vi "Launch Dynamically Load Graphics.vi"(4 "User events":T1, 6 "Template saved?":bool, 7 "Path":T2=enum."Glyphs", 8 "error in (no error)":errorcluster, 10 "button ref":refnum<vi>, 11 "animatedDecoration ref":refnum<vi>) -> (0 "error out":errorcluster)   [LabVIEW 2020]
uses:
  vi.lib/LabVIEW Icon API/lv_icon/lv_icon.lvlib
  vi.lib/LabVIEW Icon API/lv_icon/Controls/Pathes.ctl
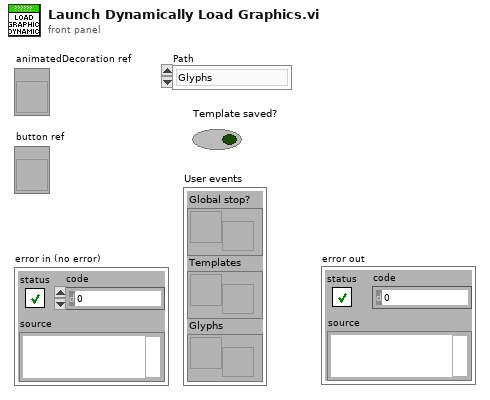
[diagram p1: front panel]
types:
  T1 = cluster{"Global stop?":refnum<user-event>, "Templates":refnum<user-event>, "Glyphs":refnum<user-event>}
  T2 = typedef "Pathes.ctl" = enum16{"Root Path", "Icon Templates", "Icon Templates VI", "Icon Templates Lib", "Glyphs"}
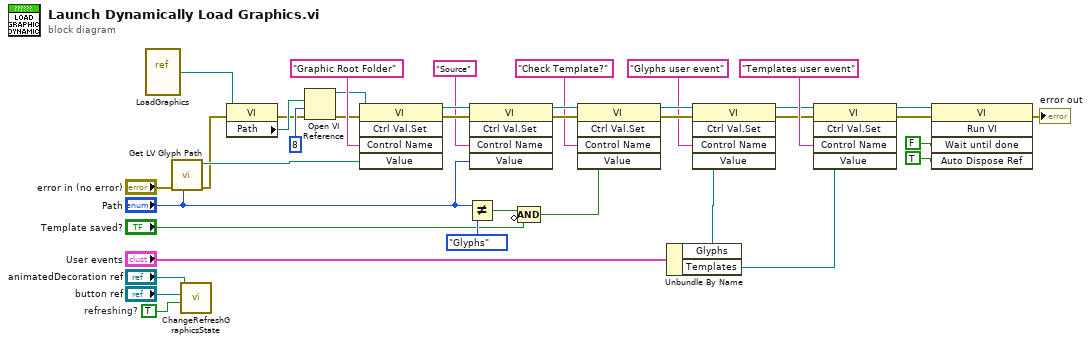
[diagram p0: block diagram]
diagram:
  w1 = TRUE  # refreshing?
  n1 = vi-ref "LoadGraphics.vi"() -> (w24:refnum<vi>)
  n2 = call "Get LV Glyph Path.vi"("Path"="Path", "error in (no error)"="error in (no error)") -> ("error out"=w18:errorcluster, "Requested Path"=w38:path)  [unwired: 1 in, 7 out]
  n3 = call "ChangeRefreshGraphicsState.vi"("refreshing?"=w1, "button ref"="button ref", "animatedDecoration ref"="animatedDecoration ref") -> ()  [unwired: 8 in, 1 out]
  n4 = property class="VI"(reference=w24, error in=w18) -> (error out=w20:errorcluster, "Path"=w23:path)  [unwired: 1 out]
  n5 = Open VI Reference(vi path=w23, options=8, error in (no error)=w20) -> (vi reference=w21:refnum<vi>, error out=w19:errorcluster)  [unwired: 3 out]
  n6 = invoke class="VI" method="Ctrl Val.Set"(reference=w21, error in=w19, "Control Name"="Graphic Root Folder", "Value"=w38) -> (reference out=w34:refnum<vi>, error out=w33:errorcluster)  [unwired: 1 in, 3 out]
  n7 = Not Equal?(x="Path", y=Pathes."Glyphs") -> (x != y?=w17:bool)
  n8 = invoke class="VI" method="Ctrl Val.Set"(reference=w34, error in=w33, "Control Name"="Source", "Value"="Path") -> (reference out=w29:refnum<vi>, error out=w28:errorcluster)  [unwired: 1 in, 3 out]
  n9 = Compound Arithmetic op=AND(w17, invert "Template saved?") -> (w15:bool)
  n10 = invoke class="VI" method="Ctrl Val.Set"(reference=w29, error in=w28, "Control Name"="Check Template?", "Value"=w15) -> (reference out=w14:refnum<vi>, error out=w13:errorcluster)  [unwired: 1 in, 3 out]
  n11 = Unbundle By Name("User events") -> ("Glyphs"=w5:refnum<user-event>, "Templates"=w4:refnum<user-event>)
  n12 = invoke class="VI" method="Ctrl Val.Set"(reference=w14, error in=w13, "Control Name"="Glyphs user event", "Value"=w5) -> (reference out=w8:refnum<vi>, error out=w7:errorcluster)  [unwired: 1 in, 3 out]
  n13 = invoke class="VI" method="Ctrl Val.Set"(reference=w8, error in=w7, "Control Name"="Templates user event", "Value"=w4) -> (reference out=w11:refnum<vi>, error out=w10:errorcluster)  [unwired: 1 in, 3 out]
  n14 = invoke class="VI" method="Run VI"(reference=w11, error in=w10, "Wait until done"=FALSE ("Wait Until Done"), "Auto Dispose Ref"=TRUE ("Auto Dispose Reference")) -> (error out=→"error out":errorcluster)  [unwired: 1 in, 4 out]
